vi "Get Build Spec XML.vi"(8 "error in":errorcluster, 11 "DOM document":refnum<k20>) -> (0 "error out":errorcluster, 2 "Build Spec XML Info":T1[](array[typedef]), 3 "DOM document out":refnum<k20>)   [LabVIEW 2020, in "Template Tool.lvlib"]
uses:
  Template Tool.lvlib
  Target XML Information.ctl
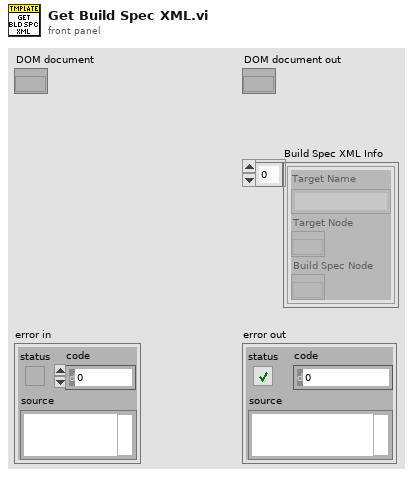
[diagram p1: front panel]
types:
  T1 = typedef "Template Tool.lvlib/Target XML Information.ctl" = cluster{"Target Name":string, "Target Node":refnum<k20>, "Build Spec Node":refnum<k20>}
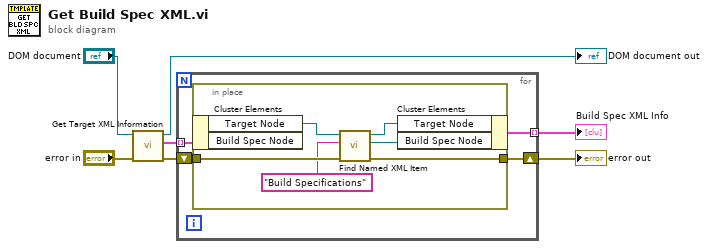
[diagram p0: block diagram]
diagram:
  n1 = call "Get Target XML Information.vi"("error in"="error in", "DOM document"="DOM document") -> ("error out"=w5:errorcluster, "target xml information"=w4:T1[], "DOM document out"=→"DOM document out":refnum<k20>)  [unwired: 7 in]
  n2 = for {
    shift-right: [w9] -> w3
    shift-left: w5 -> [w10]
    tunnel: w4 -> [w11] mode=indexing
    tunnel: [w8] -> w2 mode=indexing
    n3 = in-place {
      in-place-border: w10 -> [w17]
      in-place-border: [w14] -> w9
      n4 = in-place-cluster #1(w11) -> ("Target Node"=w16:refnum<k20>)  [unwired: 1 out]
      n5 = call "Find Named XML Item.vi"("error in"=w17, "Name"="Build Specifications", "Parent Node"=w16) -> ("error out"=w14:errorcluster, "Named Node"=w13:refnum<k20>, "Parent Node out"=w15:refnum<k20>)  [unwired: 5 in, 1 out]
      n6 = in-place-cluster #1("Target Node"=w15, "Build Spec Node"=w13) -> (w8:T1)
    }
  }
  "error out" <- w3
  "Build Spec XML Info" <- w2
